vi "OAT Output Triggered Even Angle Signal (1 Channel).vi"(0 "even-angle signal":cluster{"r0":dbl, "dr":dbl, "Y":dbl[]}={"r0"=0.0, "dr"=1.0, "Y"=[]} {"r0" format="%.2p"; "dr" format="%.2p"; "Y" format="%.2f"}, 1 "block size":i32=-1, 2 "reset? (F)":bool, 5 "even-angle channel info":T1={"channel name"="", "description"="", " channel info"={"sensor sensitivity"=1000.0, "engineering units"=1, "dB reference"=1.0, "custom label"="EU", "weighting filter"=0, "pregain"=0.0}} {"channel info"."pregain" format="%.2f"; "channel info"."weighting filter" items=["Linear", "A-weighting", "B-weighting", "C-weighting", "ITU-R 468-4", "Dolby", "CCITT", "C-message", "Wb", "Wc", "Wd", "We", "Wf", "Wh", "Wj", "Wk", "Wm", "AES17 20 kHz lowpass", "AES17 40 kHz lowpass", "AES17 20 kHz highpass", "AES17 40 kHz highpass"]; "channel info"."dB reference" format="%^.1e"; "channel info"."engineering units" items=["custom..."=0, "V"=1, "A"=21, "C"=30, "pC"=31, "s"=32, "-"=29, "Pa"=2, "N"=20, "g"=3, "m/s^2"=4, "m/s"=5, "m"=6, "mm/s"=12, "mm"=13, "micron/s"=14, "micron"=15, "in/s^2"=7, "in/s"=8, "in"=9, "mil/s"=10, "mil"=11, "rad/s^2"=16, "rad/s"=17, "rad"=18, "deg/s^2"=26, "deg/s"=27, "deg"=28, "RPM"=22, "cycle/s^2"=23, "Hz"=24, "cycle"=25, "strain"=19]; "channel info"."sensor sensitivity" format="%#_5f"}, 11 "error in (no error)":errorcluster, 12 "trigger period [rev]":dbl=1.0) -> (4 "triggered even-angle signal":cluster{"r0":dbl, "dr":dbl, "Y":dbl[]}={"r0"=0.0, "dr"=1.0, "Y"=[]} {"r0" format="%.2p"; "dr" format="%.2p"; "Y" format="%.2f"}, 6 "even-angle channel info out":T1={"channel name"="", "description"="", " channel info"={"sensor sensitivity"=1000.0, "engineering units"=1, "dB reference"=1.0, "custom label"="EU", "weighting filter"=0, "pregain"=0.0}} {"channel info"."pregain" format="%.2f"; "channel info"."weighting filter" items=["Linear", "A-weighting", "B-weighting", "C-weighting", "ITU-R 468-4", "Dolby", "CCITT", "C-message", "Wb", "Wc", "Wd", "We", "Wf", "Wh", "Wj", "Wk", "Wm", "AES17 20 kHz lowpass", "AES17 40 kHz lowpass", "AES17 20 kHz highpass", "AES17 40 kHz highpass"]; "channel info"."dB reference" format="%^.1e"; "channel info"."engineering units" items=["custom..."=0, "V"=1, "A"=21, "C"=30, "pC"=31, "s"=32, "-"=29, "Pa"=2, "N"=20, "g"=3, "m/s^2"=4, "m/s"=5, "m"=6, "mm/s"=12, "mm"=13, "micron/s"=14, "micron"=15, "in/s^2"=7, "in/s"=8, "in"=9, "mil/s"=10, "mil"=11, "rad/s^2"=16, "rad/s"=17, "rad"=18, "deg/s^2"=26, "deg/s"=27, "deg"=28, "RPM"=22, "cycle/s^2"=23, "Hz"=24, "cycle"=25, "strain"=19]; "channel info"."sensor sensitivity" format="%#_5f"}, 15 "error out":errorcluster)   [LabVIEW 2017, in "SoundVib_OAUtility.lvlib"]
doc: "Generates triggered even-angle signals for vector averaging in order power spectrum calculations. Use this VI to remove uncorrelated phenomenon for vector averaging. Each instance of this VI maintains its own state; use the N Waveforms instance of this VI to process an array of channels. Wire data to the <B>even-angle signal</B> input to determine the polymorphic instance to use or manually select the instance."
uses:
  <vilib>/addons/Sound and Vibration/Order Analysis/Utility/SoundVib_OAUtility.lvlib
  <vilib>/addons/_NISVFA/_Shared subVIs/Controls/svc_Resampled Channel Info.ctl
  <vilib>/addons/_NISVFA/_Shared subVIs/Controls/svc_Channel Info.ctl
  <vilib>/addons/_NISVFA/_Shared subVIs/Controls/svc_Engineering Units Text Ring.ctl
  <vilib>/addons/_NISVFA/_Shared subVIs/Controls/svc_Weighting Filter Text Ring.ctl
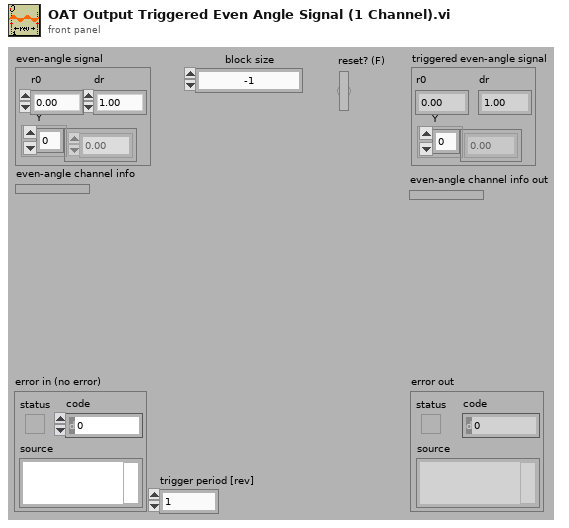
[diagram p1: front panel]
types:
  T1 = typedef "svc_Resampled Channel Info.ctl" = cluster{"channel name":string, "description":string, " channel info":T2}
  T2 = typedef "svc_Channel Info.ctl" = cluster{"sensor sensitivity":dbl, "engineering units":T3, "dB reference":dbl, "custom label":string, "weighting filter":T4, "pregain":dbl}
  T3 = typedef "svc_Engineering Units Text Ring.ctl" = u16
  T4 = typedef "svc_Weighting Filter Text Ring.ctl" = u16
  T5 = cluster{"ignore dt":bool, "ignore t0 continuity":bool, "ignore array length":bool, "ignore channel info":bool, "ignore channel name":bool}
  T6 = cluster{"r0":dbl, "dr":dbl, "even angle signal":dbl[]}
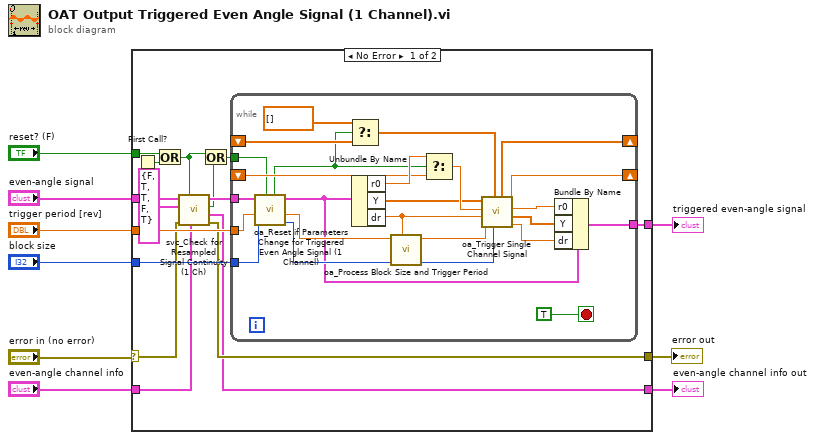
[diagram p0: block diagram]
diagram:
  n1 = case shown="No Error" "error in (no error)" {
    selector: "error in (no error)" -> [w17 w50]
    tunnel: [w24 w52] -> w9
    tunnel: "even-angle signal" -> [w23 w52]
    tunnel: "even-angle channel info" -> [w11 w51]
    tunnel: [w10 w51] -> w5
    tunnel: [w16 w50] -> w4
    tunnel: "trigger period [rev]" -> [w22 _]
    tunnel: "block size" -> [w21 _]
    tunnel: "reset? (F)" -> [w19 _]
    frame No Error {
      n2 = First Call?() -> (First Call?: T/F=w20:bool)
      n3 = Or(x=w19, y=w20) -> (x .or. y?=w15:bool)
      n4 = call <vilib>:"svc_Check for Resampled Signal Continuity (1 Ch).vi"("even angle channel info"=w11, "restart averaging (F)"=w15, "error in (no error)"=w17, "parameter controls"=T5 {"ignore dt"=FALSE, "ignore t0 continuity"=TRUE, "ignore array length"=TRUE, "ignore channel info"=FALSE, "ignore channel name"=TRUE}, "even angle signal"=w23) -> ("error out"=w16:errorcluster, "dup even angle channel info"=w10:T1, "waveform parameter changed"=w13:bool, "dup even angle signal"=w18:T6)  [unwired: 1 in, 2 out]
      n5 = Or(x=w15, y=w13) -> (x .or. y?=w14:bool)
      n6 = while {
        shift-right: [w36] -> _
        shift-left: _ -> [w47]
        shift-right: [w37] -> _
        shift-left: _ -> [w45]
        tunnel: [w39] -> w24
        tunnel: w18 -> [w27]
        tunnel: w22 -> [w31]
        tunnel: w21 -> [w29]
        tunnel: w14 -> [w25]
        stop <- TRUE stop-if-true
        n7 = call <vilib>:"oa_Reset if Parameters Change for Triggered Even Angle Signal (1 Channel).vi"("reset? (T)"=w25, "block size"=w29, "trigger period [rev]"=w31, "even angle signal"=w27) -> ("block size out"=w28:i32, "trigger period out [rev]"=w30:dbl, "even angle signal out"=w26:cluster{"r0":dbl, "dr":dbl, "Y":dbl[]}, "reset out"=w32:bool)  [unwired: 4 in]
        n8 = Select(t=dbl[] [] ("Y"), s=w32, f=w47) -> (s? t:f=w44:dbl[])
        n9 = Unbundle By Name(w26) -> ("r0"=w46:dbl, "Y"=w38:dbl[], "dr"=w34:dbl)
        n10 = call <vilib>:"oa_Process Block Size and Trigger Period.vi"("dr"=w34, "block size"=w28, "trigger period [rev]"=w30) -> ("block size out"=w35:i32, "trigger period out [rev]"=w33:dbl)  [unwired: 7 in]
        n11 = Select(t=w46, s=w32, f=w45) -> (s? t:f=w43:dbl)
        n12 = call <vilib>:"oa_Trigger Single Channel Signal.vi"("block size"=w35, "history signal"=w44, "trigger period [rev]"=w33, "dr"=w34, "history r0"=w43, "signal to be triggered"=w38) -> ("dr out"=w40:dbl, "triggered signal"=w41:dbl[], "triggered r0"=w42:dbl, "history r0"=w37:dbl, "history signal out"=w36:dbl[])  [unwired: 1 in]
        n13 = Bundle By Name(cluster=w26, "r0"=w42, "Y"=w41, "dr"=w40) -> (w39:cluster{"r0":dbl, "dr":dbl, "Y":dbl[]})
      }
    }
    frame Error {
    }
  }
  "triggered even-angle signal" <- w9
  "even-angle channel info out" <- w5
  "error out" <- w4
